vi "FCI_Lip_Symmetry_Pats.vi"(0 "Image In":T1(plugin-control), 1 "Calibrated Image":T1, 2 "Edge Options Ref ROI":T4={"Edge Polarity"=0, "Kernel Size"=3, "Width"=3, "Minimum Edge Strength"=50.0, "Interpolation Type"=enum."Zero Order", "Data Processing Method"=enum."Average"} {"Edge Polarity" items=["All Edges", "Rising Edges", "Falling Edges"]; "Minimum Edge Strength" format="%.2f"; "Width" step=2; "Kernel Size" step=2}, 3 "Line Options Ref ROI":T6={"Number of Lines"=1, "Type"=enum."First Edge Rake", "Min. Score"=10.0, "Max. Score"=1000.0, "Orientation"=0.0, "Angle Range"=70.0, "Angle Tolerance"=1.0, "Step Size"=7, "Min. SNR (db)"=0.0, "Min. Points (%)"=25.0, "Hough Iterations"=5} {"Min. Points (%)" min=0.0 max=100.0; "Min. SNR (db)" min=0.0; "Max. Score" min=0.0 max=1024.0; "Min. Score" min=0.0 max=1024.0 step=1.0}, 4 "Search Direction Ref ROI":u32, 5 "error in (no error)":errorcluster, 6 "Ref ROI":T3 {"Contours"."Type" items=["No Selection", "Point", "Line", "Rectangle", "Oval", "Polygon", "Free", "Annulus", "Unused2", "Unused3", "Broken Line", "Free Hand Line", "Rotated Rectangle"]}, 7 "Measurement ROI 1":T2 {"Contours"."Type" items=["No Selection", "Point", "Line", "Rectangle", "Oval", "Polygon", "Freehand Region", "Annulus", "Unused2", "Unused3", "Broken Line", "Freehand Line", "Rotated Rectangle"]}, 8 "Edge Options ROI 1":T4={"Edge Polarity"=0, "Kernel Size"=3, "Width"=3, "Minimum Edge Strength"=50.0, "Interpolation Type"=enum."Zero Order", "Data Processing Method"=enum."Average"} {"Edge Polarity" items=["All Edges", "Rising Edges", "Falling Edges"]; "Minimum Edge Strength" format="%.2f"; "Width" step=2; "Kernel Size" step=2}, 9 "Search Direction ROI 1":u16(ring)=2 items=["Left To Right", "Right To Left", "Top To Bottom", "Bottom To Top"], 10 "Blob Center":cluster{"Center X":dbl, "Center Y":dbl}) -> (14 "Lip Symmetry":sgl, 19 "error out":errorcluster)   [LabVIEW 2015]
uses:
  <vilib>/vision/Measure.llb/Edge Options.ctl
  <vilib>/vision/Measure.llb/Edge Polarity.ctl
  <vilib>/vision/Measure.llb/Straight Edge Options.ctl
  <vilib>/vision/Measure.llb/Straight Edge Process.ctl
  <vilib>/vision/Image Controls.llb/IMAQ Image.ctl
  SubVI/Clamp.llb/Find Min Max Position.vi
  <vilib>/vision/NI_Vision_Development_Module.lvlib
  FrameworkOverrides/Algorithm.lvclass
panel:
  out "Angle (Pixel) 2":dbl
  out "Angle (Pixel)":dbl
  out "element 4":sgl
  out "element 3":sgl
  out "element 2":sgl
  out "element":sgl
  out "Distance 2":dbl format="%.2f"
  out "Distance":dbl format="%.2f"
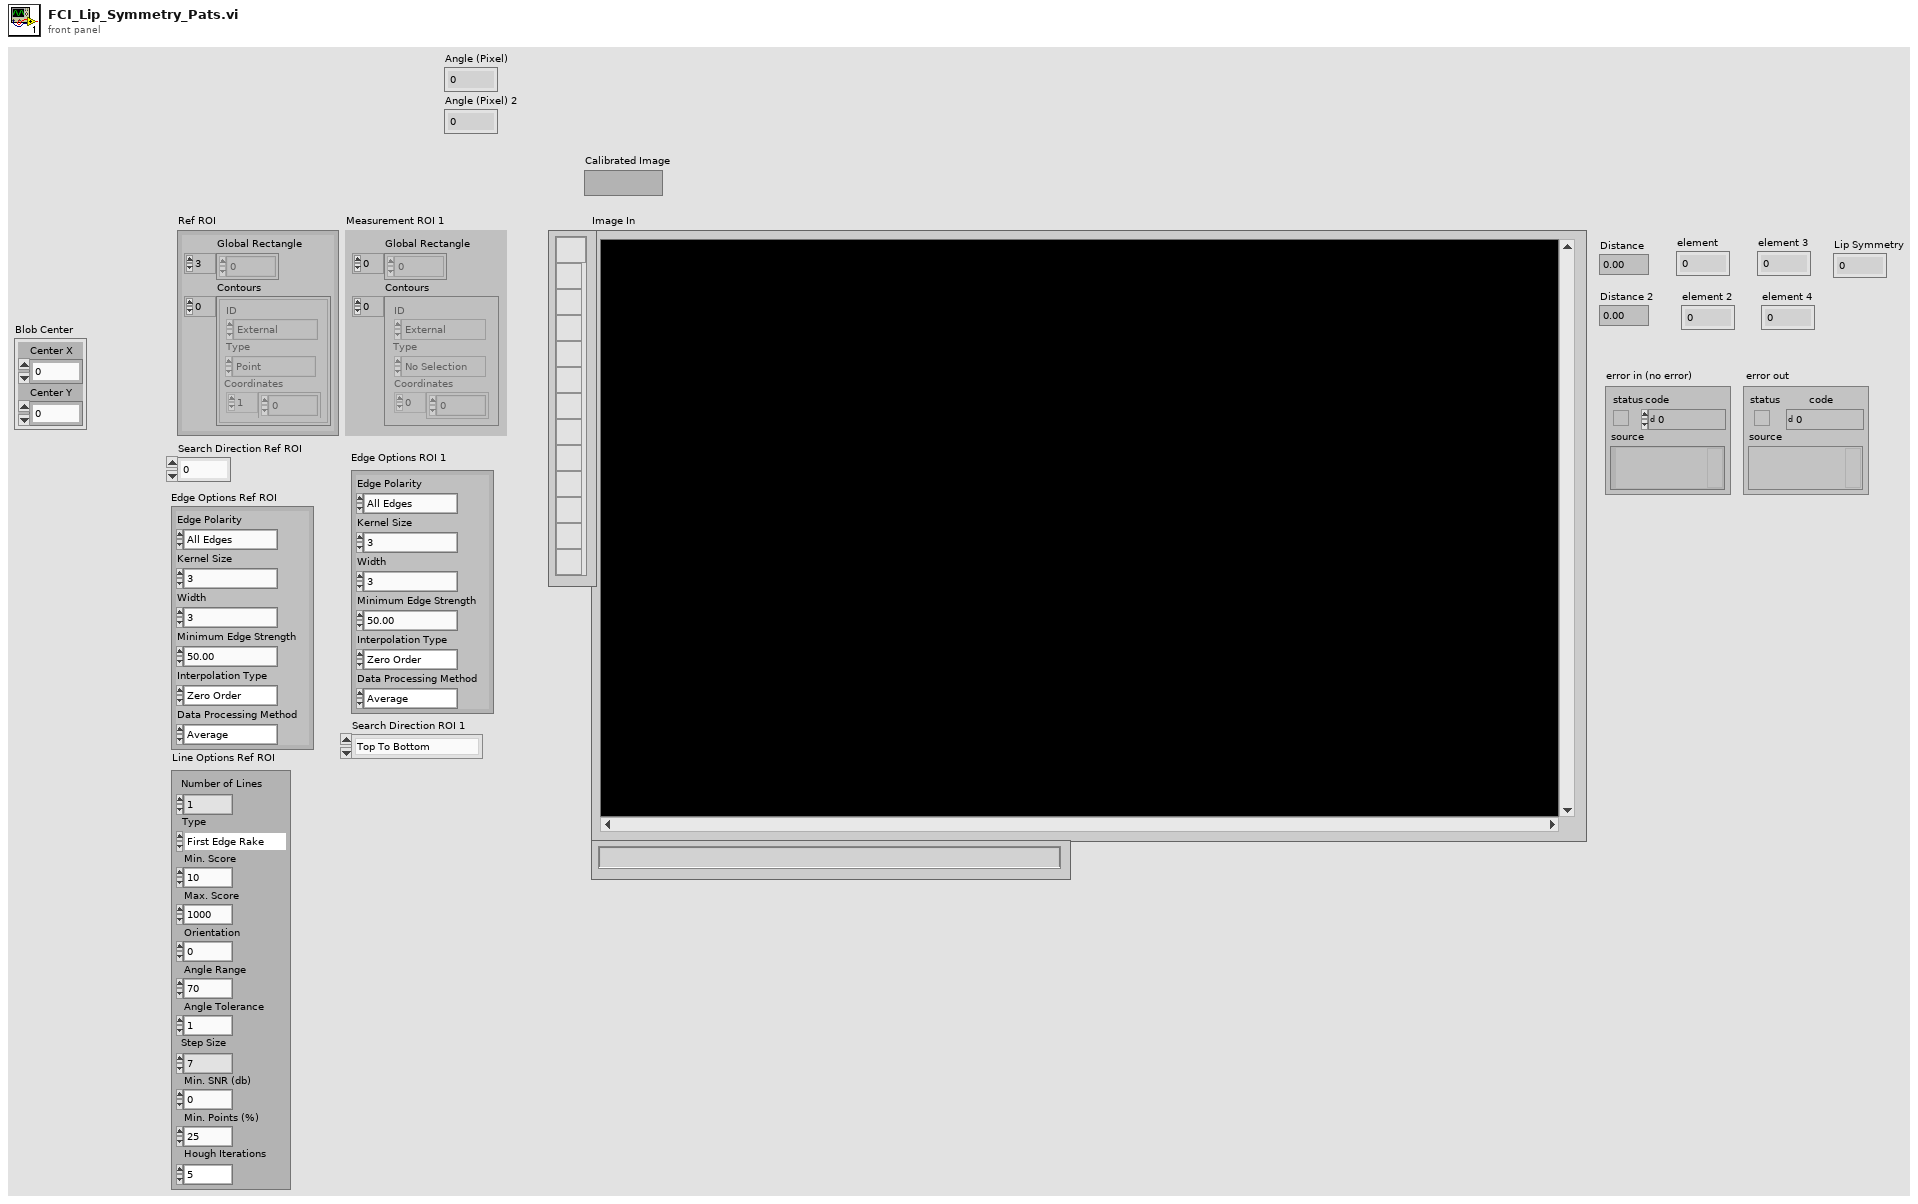
[diagram p1: front panel]
types:
  T1 = typedef "IMAQ Image.ctl" = refnum<image>
  T2 = typedef "ROI Descriptor" = cluster{"Global Rectangle":i32[], "Contours":cluster{"ID":enum32{"External", "Internal"}, "Type":u32, "Coordinates":i32[]}[]}
  T3 = cluster{"Global Rectangle":i32[], "Contours":cluster{"ID":enum32{"External", "Internal"}, "Type":u32, "Coordinates":i32[]}[]}
  T4 = typedef "Edge Options.ctl" = cluster{"Edge Polarity":T5, "Kernel Size":u32, "Width":u32, "Minimum Edge Strength":sgl, "Interpolation Type":enum32{"Zero Order", "Bilinear", "Quadratic", "Cubic", "Bilinear Fixed"}, "Data Processing Method":enum32{"Average", "Median"}}
  T5 = typedef "Edge Polarity.ctl" = u32
  T6 = typedef "Straight Edge Options.ctl" = cluster{"Number of Lines":i32, "Type":T7, "Min. Score":dbl, "Max. Score":dbl, "Orientation":dbl, "Angle Range":dbl, "Angle Tolerance":dbl, "Step Size":u32, "Min. SNR (db)":dbl, "Min. Points (%)":dbl, "Hough Iterations":i32}
  T7 = typedef "Straight Edge Process.ctl" = enum32{"First Edge Rake", "Best Edge Rake", "Hough Edge Rake", "First Edge Projection", "Best Edge Projection"}
  T8 = typedef "IMAQ Rectangle" = cluster{"Left":i32, "Top":i32, "Right":i32, "Bottom":i32, "Rotation":dbl}
  T9 = cluster{"Search Direction":u32, "Edge Options":T4, "Show Search Area":bool, "Show Search Lines":bool, "Show Edges Found":bool, "Show Result":bool, "Search Area Color":u32, "Search Lines Color":u32, "Edge Locations Color":u32, "Result Color":u32, "Overlay Group Name":string}
  T10 = cluster{"Left":dbl, "Top":dbl, "Right":dbl, "Bottom":dbl, "Angle":dbl}
  T11 = cluster{"Left":i32, "Top":i32, "Right":i32, "Bottom":i32, "Angle":dbl}
  T12 = cluster{"Point1 (Pixels)":cluster{"X":sgl, "Y":sgl}, "Point2 (Pixels)":cluster{"X":sgl, "Y":sgl}, "Point1 (Real-World)":cluster{"X":sgl, "Y":sgl}, "Point2 (Real-World)":cluster{"X":sgl, "Y":sgl}, "Angle (Pixel)":dbl, "Angle (Real-World)":dbl, "Score":dbl, "Straightness":dbl, "Average SNR (db)":dbl, "Calibration Valid":bool}[]
  T13 = cluster{"Point1 (Pixels)":cluster{"X":sgl, "Y":sgl}, "Point2 (Pixels)":cluster{"X":sgl, "Y":sgl}, "Point1 (Real-World)":cluster{"X":sgl, "Y":sgl}, "Point2 (Real-World)":cluster{"X":sgl, "Y":sgl}, "Angle (Pixel)":dbl, "Angle (Real-World)":dbl, "Score":dbl, "Straightness":dbl, "Average SNR (db)":dbl, "Calibration Valid":bool}
  T14 = cluster{"Point1 (Pixels)":cluster{"X":sgl, "Y":sgl}, "Point2 (Pixels)":cluster{"X":sgl, "Y":sgl}}
  T15 = cluster{"Point 1":cluster{"X":sgl, "Y":sgl}, "Point 2":cluster{"X":sgl, "Y":sgl}}
  T16 = cluster{cluster{"X":sgl, "Y":sgl}, cluster{"X":sgl, "Y":sgl}}[]
  T17 = cluster{cluster{"X":sgl, "Y":sgl}, cluster{"X":sgl, "Y":sgl}}
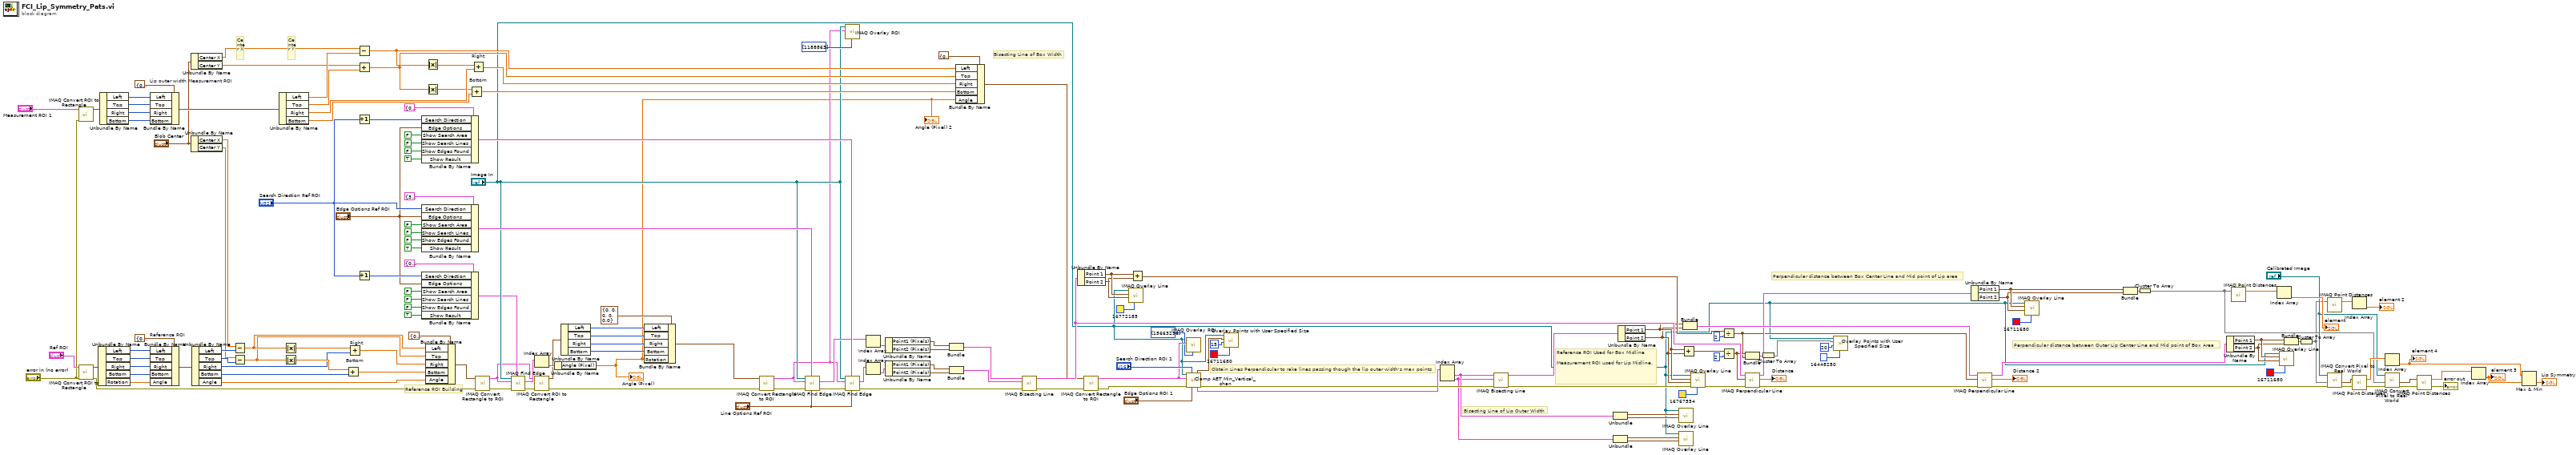
[diagram p0: block diagram]
diagram:
  # "Center Y"
  # "Center X"
  # "Reference ROI Building"
  # "Reference ROI Used for Box Midline\n\nMeasurement ROI used for Lip Midline."
  # "Perpendicular distance between Outer Lip Center Line and Mid point of Box Area"
  # "Perpendicular distance between Box Center Line and Mid point of Lip area"
  # "Bisecting Line of Lip Outer Width"
  # "Bisecting Line of Box Width"
  # "Obtain Lines Perpendicular to rake lines passing though the lip outer width's max points"
  n1 = call "IMAQ Convert ROI to Rectangle"("error in (no error)"="error in (no error)", "ROI Descriptor"="Measurement ROI 1") -> ("Rectangle"=w39:T8)  [unwired: 7 in, 1 out]
  n2 = call "IMAQ Convert ROI to Rectangle"("error in (no error)"="error in (no error)", "ROI Descriptor"="Ref ROI") -> ("error out"=w56:errorcluster, "Rectangle"=w62:T8)  [unwired: 7 in]
  n3 = Unbundle By Name(w62) -> ("Left"=w60:i32, "Top"=w59:i32, "Right"=w58:i32, "Bottom"=w57:i32, "Rotation"=w61:dbl)
  n4 = Unbundle By Name(w39) -> ("Left"=w38:i32, "Top"=w37:i32, "Right"=w36:i32, "Bottom"=w35:i32)
  n5 = Bundle By Name "Lip outer width Measurement ROI"(cluster=T10 {"Left"=0.0, "Top"=0.0, "Right"=0.0, "Bottom"=0.0, "Angle"=0.0} ("input cluster"), "Left"=w38, "Top"=w37, "Right"=w36, "Bottom"=w35) -> (w42:T10)
  n6 = Bundle By Name "Reference ROI"(cluster=T11 {"Left"=0, "Top"=0, "Right"=0, "Bottom"=0, "Angle"=0.0} ("input cluster"), "Left"=w60, "Top"=w59, "Right"=w58, "Bottom"=w57, "Angle"=w61) -> (w66:T11)
  n7 = Unbundle By Name("Blob Center") -> ("Center X"=w41:dbl, "Center Y"=w40:dbl)
  n8 = Unbundle By Name("Blob Center") -> ("Center X"=w64:dbl, "Center Y"=w63:dbl)
  n9 = Unbundle By Name(w66) -> ("Left"=w73:i32, "Top"=w72:i32, "Right"=w71:i32, "Bottom"=w70:i32, "Angle"=w69:dbl)
  n10 = Subtract(x=w64, y=w73) -> (x-y=w77:dbl)
  n11 = Subtract(x=w63, y=w72) -> (x-y=w76:dbl)
  n12 = Unbundle By Name(w42) -> ("Left"=w49:dbl, "Top"=w48:dbl, "Right"=w47:dbl, "Bottom"=w46:dbl)
  n13 = Absolute Value(x=w77) -> (abs(x)=w80:dbl)
  n14 = Absolute Value(x=w76) -> (abs(x)=w79:dbl)
  n15 = Add "Bottom"(x=w79, y=w70) -> (x+y=w74:dbl)
  n16 = Add "Right"(x=w80, y=w71) -> (x+y=w75:dbl)
  n17 = Subtract(x=w41, y=w49) -> (x-y=w52:dbl)
  n18 = Add(x=w40, y=w48) -> (x+y=w44:dbl)
  n19 = Increment(x="Search Direction Ref ROI") -> (x+1=w97:u32)
  n20 = Increment(x="Search Direction Ref ROI") -> (x+1=w22:u32)
  n21 = Bundle By Name(cluster=T9 {"Search Direction"=0, "Edge Options"={"Edge Polarity"=0, "Kernel Size"=3, "Width"=3, "Minimum Edge Strength"=10.0, "Interpolation Type"=enum."Bilinear Fixed", "Data Processing Method"=enum."Average"}, "Show Search Area"=FALSE, "Show Search Lines"=FALSE, "Show Edges Found"=FALSE, "Show Result"=TRUE, "Search Area Color"=65280, "Search Lines Color"=255, "Edge Locations Color"=16776960, "Result Color"=16711680, "Overlay Group Name"=""} ("Options"), "Search Direction"=w97, "Edge Options"="Edge Options Ref ROI", "Show Search Area"=FALSE, "Show Search Lines"=FALSE, "Show Edges Found"=FALSE, "Show Result"=TRUE) -> (w160:T9)
  n22 = Bundle By Name(cluster=T9 {"Search Direction"=3, "Edge Options"={"Edge Polarity"=0, "Kernel Size"=3, "Width"=3, "Minimum Edge Strength"=50.0, "Interpolation Type"=enum."Bilinear Fixed", "Data Processing Method"=enum."Average"}, "Show Search Area"=FALSE, "Show Search Lines"=FALSE, "Show Edges Found"=FALSE, "Show Result"=TRUE, "Search Area Color"=65280, "Search Lines Color"=255, "Edge Locations Color"=16776960, "Result Color"=16711680, "Overlay Group Name"=""} ("Options"), "Search Direction"="Search Direction Ref ROI", "Edge Options"="Edge Options Ref ROI", "Show Search Area"=FALSE, "Show Search Lines"=FALSE, "Show Edges Found"=FALSE, "Show Result"=TRUE) -> (w167:T9)
  n23 = Bundle By Name(cluster=T9 {"Search Direction"=0, "Edge Options"={"Edge Polarity"=0, "Kernel Size"=3, "Width"=3, "Minimum Edge Strength"=10.0, "Interpolation Type"=enum."Bilinear Fixed", "Data Processing Method"=enum."Average"}, "Show Search Area"=FALSE, "Show Search Lines"=FALSE, "Show Edges Found"=FALSE, "Show Result"=TRUE, "Search Area Color"=65280, "Search Lines Color"=255, "Edge Locations Color"=16776960, "Result Color"=16711680, "Overlay Group Name"=""} ("Options"), "Search Direction"=w22, "Edge Options"="Edge Options Ref ROI", "Show Search Area"=FALSE, "Show Search Lines"=FALSE, "Show Edges Found"=FALSE, "Show Result"=TRUE) -> (w20:T9)
  n24 = Absolute Value(x=w52) -> (abs(x)=w54:dbl)
  n25 = Absolute Value(x=w44) -> (abs(x)=w45:dbl)
  n26 = Bundle By Name(cluster=T10 {"Left"=0.0, "Top"=0.0, "Right"=0.0, "Bottom"=0.0, "Angle"=0.0} ("input cluster"), "Left"=w77, "Top"=w76, "Right"=w75, "Bottom"=w74, "Angle"=w69) -> (w68:T10)
  n27 = Add "Bottom"(x=w45, y=w46) -> (x+y=w50:dbl)
  n28 = Add "Right"(x=w54, y=w47) -> (x+y=w51:dbl)
  n29 = call "IMAQ Convert Rectangle to ROI"("error in (no error)"=w56, "Rectangle"=w68) -> ("error out"=w17:errorcluster, "ROI Descriptor"=w13:T2)  [unwired: 7 in]
  n30 = call "IMAQ Find Edge"("Options"=w20, "error in (no error)"=w17, "ROI Descriptor"=w13, "Image"="Image In") -> ("error out"=w12:errorcluster, "Straight Edges"=w19:T12)  [unwired: 4 in, 2 out]
  n31 = Index Array(array=w19) -> (element=w18:T13)  [unwired: 1 in]
  n32 = call "IMAQ Convert ROI to Rectangle"("error in (no error)"=w12, "ROI Descriptor"=w13) -> ("error out"=w6:errorcluster, "Rectangle"=w11:T8)  [unwired: 7 in]
  n33 = Unbundle By Name(w18) -> ("Angle (Pixel)"=w4:dbl)
  "Angle (Pixel)" <- w4
  "Angle (Pixel) 2" <- w4
  n34 = Unbundle By Name(w11) -> ("Left"=w10:i32, "Top"=w9:i32, "Right"=w8:i32, "Bottom"=w7:i32)
  n35 = Bundle By Name(cluster=T8 {"Left"=0, "Top"=0, "Right"=0, "Bottom"=0, "Rotation"=0.0} ("Rectangle"), "Left"=w10, "Top"=w9, "Right"=w8, "Bottom"=w7, "Rotation"=w4) -> (w15:T8)
  n36 = call "IMAQ Convert Rectangle to ROI"("error in (no error)"=w6, "Rectangle"=w15) -> ("error out"=w5:errorcluster, "ROI Descriptor"=w14:T2)  [unwired: 7 in]
  n37 = call "IMAQ Find Edge"("Line Fit Options"="Line Options Ref ROI", "Options"=w167, "error in (no error)"=w5, "ROI Descriptor"=w14, "Image"="Image In") -> ("error out"=w166:errorcluster, "Straight Edges"=w159:T12)  [unwired: 3 in, 2 out]
  n38 = call "IMAQ Overlay ROI"("Colors (Green)"=u32[] [1188863], "ROI Descriptor"=w14, "Image"="Image In") -> ()  [unwired: 7 in, 2 out]
  n39 = call "IMAQ Find Edge"("Line Fit Options"="Line Options Ref ROI", "Options"=w160, "error in (no error)"=w166, "ROI Descriptor"=w14, "Image"="Image In") -> ("error out"=w149:errorcluster, "Straight Edges"=w158:T12)  [unwired: 3 in, 2 out]
  n40 = Index Array(array=w159) -> (element=w157:T13)  [unwired: 1 in]
  n41 = Index Array(array=w158) -> (element=w156:T13)  [unwired: 1 in]
  n42 = Unbundle By Name(w157) -> ("Point1 (Pixels)"=w155:cluster{"X":sgl, "Y":sgl}, "Point2 (Pixels)"=w154:cluster{"X":sgl, "Y":sgl})
  n43 = Unbundle By Name(w156) -> ("Point1 (Pixels)"=w153:cluster{"X":sgl, "Y":sgl}, "Point2 (Pixels)"=w152:cluster{"X":sgl, "Y":sgl})
  n44 = Bundle("Point1 (Pixels)"=w155, "Point2 (Pixels)"=w154) -> (w151:T14)  [unwired: 1 in]
  n45 = Bundle("Point1 (Pixels)"=w153, "Point2 (Pixels)"=w152) -> (w150:T14)  [unwired: 1 in]
  n46 = Bundle By Name(cluster=T10 {"Left"=0.0, "Top"=0.0, "Right"=0.0, "Bottom"=0.0, "Angle"=0.0} ("input cluster"), "Left"=w52, "Top"=w44, "Right"=w51, "Bottom"=w50, "Angle"=w4) -> (w30:T10)
  n47 = call "IMAQ Bisecting Line"("error in (no error)"=w149, "Line 2"=w150, "Line 1"=w151) -> ("error out"=w31:errorcluster, "Bisecting Line"=w133:T15)  [unwired: 7 in]
  n48 = Unbundle By Name(w133) -> ("Point 1"=w127:cluster{"X":sgl, "Y":sgl}, "Point 2"=w126:cluster{"X":sgl, "Y":sgl})
  n49 = call "IMAQ Convert Rectangle to ROI"("error in (no error)"=w31, "Rectangle"=w30) -> ("error out"=w147:errorcluster, "ROI Descriptor"=w103:T2)  [unwired: 7 in]
  n50 = call "IMAQ Overlay Line"("Color"=u32 16772185, "End Point"=w126, "Start Point"=w127, "Image"="Image In") -> ()  [unwired: 6 in, 2 out]
  n51 = Add(x=w127, y=w126) -> (x+y=w125:cluster{"X":sgl, "Y":sgl})
  n52 = call "IMAQ Overlay ROI"("Colors (Green)"=u32[] [15663296], "ROI Descriptor"=w103, "Image"="Image In") -> ()  [unwired: 7 in, 2 out]
  n53 = call "Clamp AET Min_Vertical_shan.vi"("Image"="Image In", "Scanning axis"="Search Direction ROI 1", "ROI Descriptor"=w103, "error in (no error)"=w147, "Edge Options"="Edge Options ROI 1") -> ("Edge Coordinates"=w100:cluster{"X":sgl, "Y":sgl}[], "Perpendicular Lines"=w144:T16, "error out"=w143:errorcluster)  [unwired: 3 in, 5 out]
  n54 = call "Overlay Points with User Specified Size.vi"("Color"=u32 16711680, "Point Diameter (5)"=u32 15, "Points"=w100, "Image In"="Image In") -> ()  [unwired: 6 in, 2 out]
  n55 = Index Array(array=w144) -> (element #1=w139:T17, element #2=w136:T17)  [unwired: 2 in]
  n56 = call "IMAQ Bisecting Line"("error in (no error)"=w143, "Line 2"=w136, "Line 1"=w139) -> ("error out"=w141:errorcluster, "Bisecting Line"=w142:T15)  [unwired: 7 in]
  n57 = Unbundle(w139) -> (w138:cluster{"X":sgl, "Y":sgl}, w137:cluster{"X":sgl, "Y":sgl})
  n58 = Unbundle(w136) -> (w135:cluster{"X":sgl, "Y":sgl}, w134:cluster{"X":sgl, "Y":sgl})
  n59 = Unbundle By Name(w142) -> ("Point 1"=w124:cluster{"X":sgl, "Y":sgl}, "Point 2"=w123:cluster{"X":sgl, "Y":sgl})
  n60 = call "IMAQ Overlay Line"("End Point"=w137, "Start Point"=w138, "Image"="Image In") -> ()  [unwired: 7 in, 2 out]
  n61 = call "IMAQ Overlay Line"("End Point"=w134, "Start Point"=w135, "Image"="Image In") -> ()  [unwired: 7 in, 2 out]
  n62 = Add(x=w124, y=w123) -> (x+y=w132:cluster{"X":sgl, "Y":sgl})
  n63 = Bundle("Point 1"=w124, "Point 2"=w123) -> (w122:T15)  [unwired: 1 in]
  n64 = call "IMAQ Overlay Line"("Color"=u32 16767554, "error in (no error)"=w141, "End Point"=w123, "Start Point"=w124, "Image"="Image In") -> ("error out"=w96:errorcluster)  [unwired: 5 in, 1 out]
  n65 = Divide(x=w125, y=2) -> (x/y=w83:cluster{"X":sgl, "Y":sgl})
  n66 = Divide(x=w132, y=2) -> (x/y=w84:cluster{"X":sgl, "Y":sgl})
  n67 = Bundle(w84, w83) -> (w82:T17)  [unwired: 1 in]
  n68 = call "IMAQ Perpendicular Line"("error in (no error)"=w96, "Point"=w84, "Line"=w133) -> ("error out"=w94:errorcluster, "Distance"=→"Distance":dbl, "Perpendicular Line"=w118:T15)  [unwired: 6 in]
  n69 = Cluster To Array(cluster=w82) -> (array=w1:cluster{"X":sgl, "Y":sgl}[])
  n70 = call "Overlay Points with User Specified Size.vi"("Color"=u32 16448250, "Point Diameter (5)"=u32 20, "Points"=w1, "Image In"="Image In") -> ()  [unwired: 6 in, 2 out]
  n71 = Unbundle By Name(w118) -> ("Point 1"=w117:cluster{"X":sgl, "Y":sgl}, "Point 2"=w116:cluster{"X":sgl, "Y":sgl})
  n72 = call "IMAQ Perpendicular Line"("error in (no error)"=w94, "Point"=w83, "Line"=w122) -> ("error out"=w92:errorcluster, "Distance"=→"Distance 2":dbl, "Perpendicular Line"=w121:T15)  [unwired: 6 in]
  n73 = call "IMAQ Overlay Line"("Color"=u32 16711680, "End Point"=w116, "Start Point"=w117, "Image"="Image In") -> ()  [unwired: 6 in, 2 out]
  n74 = Bundle("Point 1"=w117, "Point 2"=w116) -> (w108:T15)  [unwired: 1 in]
  n75 = Cluster To Array(cluster=w108) -> (array=w3:cluster{"X":sgl, "Y":sgl}[])
  n76 = Unbundle By Name(w121) -> ("Point 1"=w115:cluster{"X":sgl, "Y":sgl}, "Point 2"=w114:cluster{"X":sgl, "Y":sgl})
  n77 = call "IMAQ Point Distances"("Points"=w3) -> ("Distances"=w113:sgl[])  [unwired: 4 in, 1 out]
  n78 = Index Array(array=w113) -> (element=→"element":sgl)  [unwired: 1 in]
  n79 = call "IMAQ Overlay Line"("Color"=u32 16711680, "End Point"=w114, "Start Point"=w115, "Image"="Image In") -> ()  [unwired: 6 in, 2 out]
  n80 = Bundle("Point 1"=w115, "Point 2"=w114) -> (w109:T15)  [unwired: 1 in]
  n81 = Cluster To Array(cluster=w109) -> (array=w2:cluster{"X":sgl, "Y":sgl}[])
  n82 = call "IMAQ Point Distances"("Points"=w2) -> ("Distances"=w110:sgl[])  [unwired: 4 in, 1 out]
  n83 = call "IMAQ Convert Pixel to Real World"("error in (no error)"=w92, "Array of Pixel Coordinates"=w2, "Calibrated Image"="Calibrated Image") -> ("error out"=w93:errorcluster, "Array of Real World Coordinates"=w107:cluster{"X":sgl, "Y":sgl}[])  [unwired: 3 in, 4 out]
  n84 = Index Array(array=w110) -> (element=→"element 2":sgl)  [unwired: 1 in]
  n85 = call "IMAQ Point Distances"("Points"=w107, "error in (no error)"=w93) -> ("Distances"=w104:sgl[], "error out"=w91:errorcluster)  [unwired: 3 in]
  n86 = call "IMAQ Convert Pixel to Real World"("error in (no error)"=w91, "Array of Pixel Coordinates"=w3, "Calibrated Image"="Calibrated Image") -> ("error out"=w90:errorcluster, "Array of Real World Coordinates"=w106:cluster{"X":sgl, "Y":sgl}[])  [unwired: 3 in, 4 out]
  n87 = Index Array(array=w104) -> (element=w89:sgl)  [unwired: 1 in]
  "element 4" <- w89
  n88 = call "IMAQ Point Distances"("Points"=w106, "error in (no error)"=w90) -> ("Distances"=w105:sgl[], "error out"=→"error out":errorcluster)  [unwired: 3 in]
  n89 = Index Array(array=w105) -> (element=w88:sgl)  [unwired: 1 in]
  "element 3" <- w88
  n90 = Max & Min(x=w89, y=w88) -> (min(x,y)=→"Lip Symmetry":sgl)  [unwired: 1 out]
